vi "Write RunID.vi"(8 "error in (no error)":errorcluster, 10 "RunID":string, 11 "AnalysisListItems in":refnum<class "AnalysisListItems.lvclass">) -> (0 "error out":errorcluster, 3 "AnalysisListItems out":refnum<class "AnalysisListItems.lvclass">)   [LabVIEW 2018, in "AnalysisListItems.lvclass"]
uses:
  AnalysisListItems.lvclass
  AnalysisListItems.lvclass/AnalysisListItems.ctl
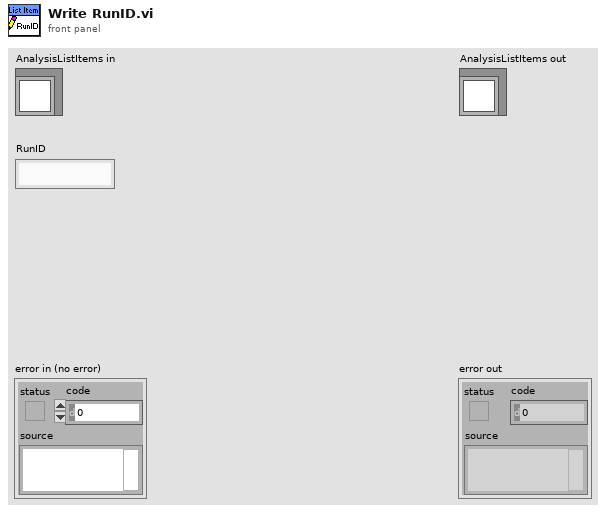
[diagram p1: front panel]
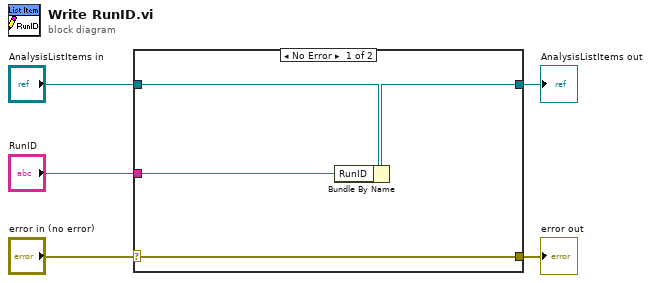
[diagram p0: block diagram]
diagram:
  n1 = case shown="No Error" "error in (no error)" {
    selector: "error in (no error)" -> [w9 w10]
    tunnel: [w9 w10] -> w4
    tunnel: [w7 w11] -> w2
    tunnel: "AnalysisListItems in" -> [w8 w11]
    tunnel: "RunID" -> [w6 _]
    frame No Error {
      n2 = Bundle By Name(cluster=w8, "RunID"=w6) -> (w7:refnum<class "AnalysisListItems.lvclass">)
    }
    frame Error {
    }
  }
  "error out" <- w4
  "AnalysisListItems out" <- w2
